vi "MISC Basic Find and Replace.vi"(8 "Case Sensitive (T)":bool=TRUE, 9 "Replace Text":string, 10 "Search Text":string, 11 "Input String":string) -> (2 "Matches":i32, 3 "Output String":string)   [LabVIEW 2012]
doc: "This routine searches the input string for the string contained in \"Search String\" and, if found, replaces all instances of \"Search String\" with the \"Replace String\"."
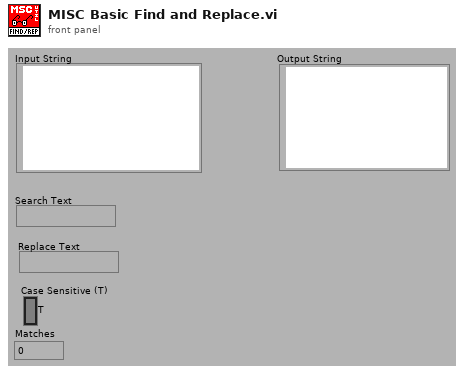
[diagram p1: front panel]
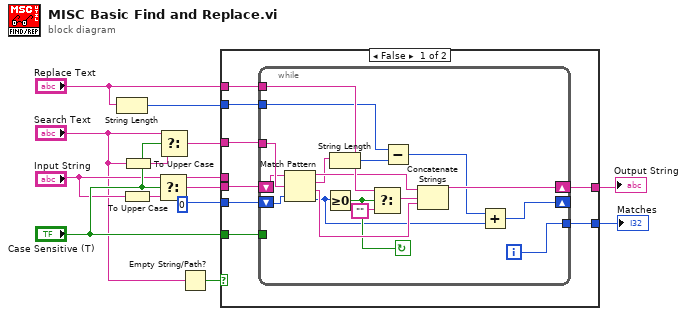
[diagram p0: block diagram]
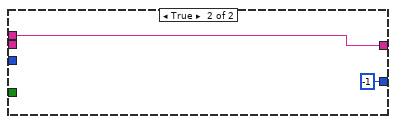
[diagram p2: hidden frame]
diagram:
  n1 = String Length(string="Replace Text") -> (length=w4:i32)
  n2 = To Upper Case(1:"Input String") -> (0:w13:string)
  n3 = To Upper Case(1:"Search Text") -> (0:w8:string)
  n4 = Select(t="Input String", s="Case Sensitive (T)", f=w13) -> (s? t:f=w12:string)
  n5 = Select(t="Search Text", s="Case Sensitive (T)", f=w8) -> (s? t:f=w10:string)
  n6 = Empty String/Path?(string/path="Search Text") -> (empty?=w3:bool)
  n7 = case shown="False" w3 {
    tunnel: w12 -> [w21 _]
    tunnel: [w20 w40] -> w11
    tunnel: w10 -> [w19 _]
    tunnel: "Case Sensitive (T)" -> [w18 _]
    tunnel: [w17 -1 ("offset past match")] -> w7
    tunnel: 0 -> [w16 _]
    tunnel: "Replace Text" -> [w15 _]
    tunnel: w4 -> [w14 _]
    tunnel: "Input String" -> [_ w40]
    frame False {
      n8 = while {
        tunnel: w14 -> [w28]
        shift-left: w16 -> [w30]
        shift-right: [w25] -> _
        tunnel: [w22] -> w17
        shift-left: w21 -> [w32]
        shift-right: [w31] -> w20
        tunnel: w18 -> [_]
        tunnel: w15 -> [w37]
        tunnel: w19 -> [w38]
        i -> [w22]
        stop <- w24 continue-if-true
        n9 = Match Pattern(string=w32, regular expression=w38, offset (0)=w30) -> (before substring=w35:string, match substring=w29:string, after substring=w33:string, offset past match=w23:i32)
        n10 = Greater Or Equal To 0?(x=w23) -> (x >= 0?=w24:bool)
        n11 = String Length(string=w29) -> (length=w27:i32)
        n12 = Select(t=w37, s=w24, f="") -> (s? t:f=w34:string)
        n13 = Subtract(x=w28, y=w27) -> (x-y=w26:i32)
        n14 = Concatenate Strings(w35, w34, w33) -> (w31:string)
        n15 = Add(x=w26, y=w23) -> (x+y=w25:i32)
      }
    }
    frame True {
    }
  }
  "Output String" <- w11
  "Matches" <- w7
